vi "Error_Handle No Set Can Value.vi"(5 "Max # Of Tries":i32=5, 7 "Loop Itteration":i32, 10 "Previous Error":errorcluster, 11 "Error":errorcluster) -> (2 "Stop Out":bool, 3 "Error Out":errorcluster)   [LabVIEW 2023]
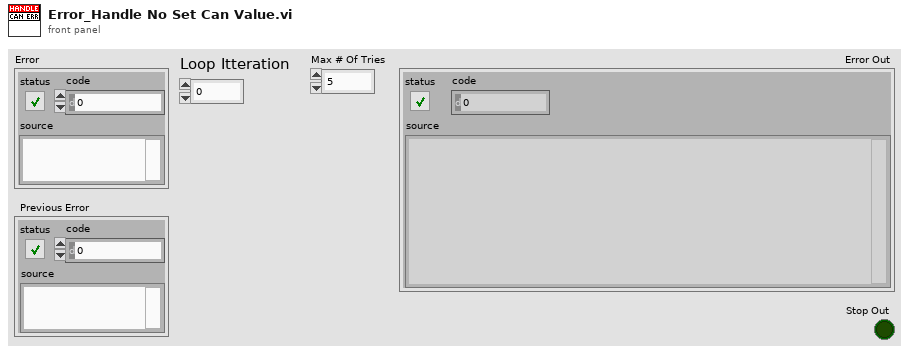
[diagram p1: front panel]
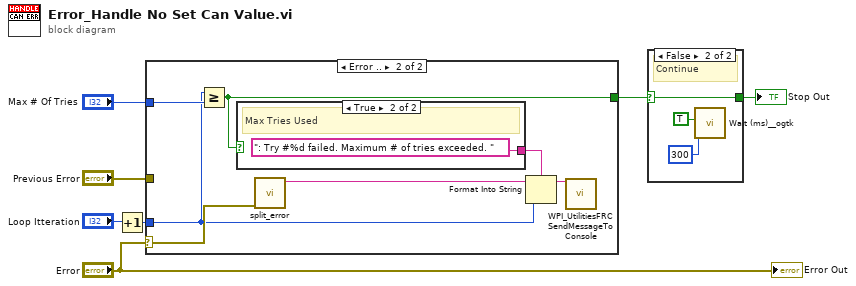
[diagram p0: block diagram]
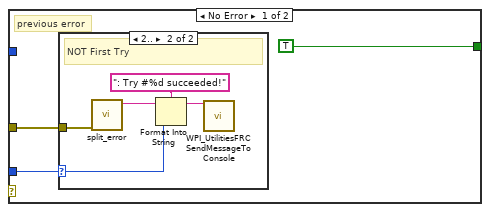
[diagram p3: hidden frame]
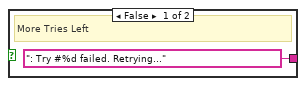
[diagram p5: hidden frame]
diagram:
  n1 = Increment(x="Loop Itteration") -> (x+1=w7:i32)
  n2 = case shown="Error .." "Error" {
    selector: "Error" -> [_ w21]
    tunnel: [TRUE ("stop") w18] -> w5
    tunnel: "Previous Error" -> [w9 _]
    tunnel: w7 -> [w8 w16]
    tunnel: "Max # Of Tries" -> [_ w17]
    frame No Error {
      # "previous error"
      n3 = case shown="2.." w8 {
        selector: w8 -> [_ w11]
        tunnel: w9 -> [_ w14]
        frame ..1 {
          # "First Try"
        }
        frame 2.. {
          # "NOT First Try"
          n4 = call "split_error.vi"("error in"=w14) -> ("Details"=w13:string)  [unwired: 7 in, 3 out]
          n5 = Format Into String(format string=": Try #%d succeeded!" ("message"), initial string=w13, w11) -> (resulting string=w12:string)  [unwired: 1 in, 1 out]
          n6 = call <vilib>:"WPI_UtilitiesFRC SendMessageToConsole.vi"("Message"=w12) -> ()  [unwired: 14 in, 1 out]
        }
      }
    }
    frame Error {
      n7 = Greater Or Equal?(x=w16, y=w17) -> (x >= y?=w18:bool)
      n8 = case shown="True" w18 {
        tunnel: [": Try #%d failed. Retrying..." ("message") ": Try #%d failed. Maximum # of tries exceeded. " ("message")] -> w22
        frame False {
          # "More Tries Left"
        }
        frame True {
          # "Max Tries Used"
        }
      }
      n9 = call "split_error.vi"("error in"=w21) -> ("Details"=w20:string)  [unwired: 7 in, 3 out]
      n10 = Format Into String(format string=w22, initial string=w20, w16) -> (resulting string=w19:string)  [unwired: 1 in, 1 out]
      n11 = call <vilib>:"WPI_UtilitiesFRC SendMessageToConsole.vi"("Message"=w19) -> ()  [unwired: 14 in, 1 out]
    }
  }
  n12 = case shown="False" w5 {
    selector: w5 -> [w25 w27]
    tunnel: [w25 w27] -> w4
    frame True {
      # "Stop"
    }
    frame False {
      # "Continue"
      n13 = call "Wait (ms)__ogtk.vi"("Wait on Error (FALSE)"=TRUE, "milliseconds to wait"=u32 300 ("Retry Delay (ms)")) -> ()  [unwired: 8 in, 2 out]
    }
  }
  "Stop Out" <- w4
  "Error Out" <- "Error"
